vi "IrDA Date Server.vi"() -> ()   [LabVIEW 2013]
doc: "Sends the current time and date via TCP to all Date Client VIs that connect to it. This VI has two parts -- a loop that listens for each client to connect, and a loop that sends the date and time to each connection in the queue."
panel:
  in  "listen halted":bool
  in  "stop":bool
  out "# connections":i32
  in  "empty":refnum<k19>[](array[refnum])
  in  "empty":refnum<k19>[](array[refnum])
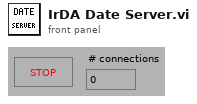
[diagram p1: front panel]
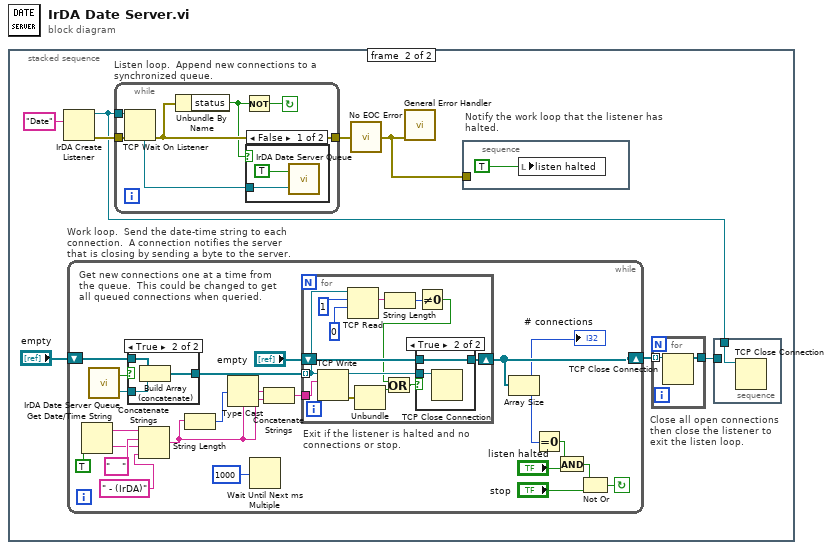
[diagram p0: block diagram]
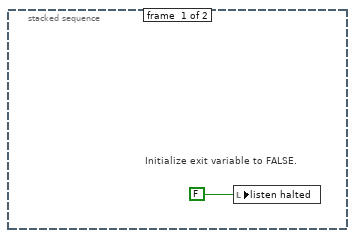
[diagram p2: hidden frame]
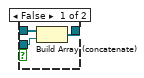
[diagram p3: hidden frame]
diagram:
  n1 = stacked-sequence {
    frame #0 {
      # "Initialize exit variable to FALSE."
      n2 = local write "listen halted"(FALSE) -> ()
    }
    frame #1 {
      # "Close all open connections then close the listener to exit the listen loop."
      # "Notify the work loop that the listener has halted."
      n3 = IrDA Create Listener(10:"Date" ("service name")) -> (0:w6:errorcluster, 3:w5:refnum<k19>)  [unwired: 1 in]
      n4 = while "Work loop.  Send the date-time string to each connection.  A connection notifies the server that is closing by sending a byte to the server." {
        shift-left: "empty" -> [w29]
        shift-right: [w20] -> w8
        stop <- w12 continue-if-true
        # "Get new connections one at a time from the queue.  This could be changed to get all queued connections when queried."
        # "Exit if the listener is halted and no connections or stop."
        n5 = Get Date/Time String(want seconds? (F)=TRUE) -> (date string=w25:string, time string=w17:string)  [unwired: 2 out]
        n6 = call "IrDA Date Server Queue.vi"() -> ("value"=w31:refnum<k19>, "valid?"=w30:bool)  [unwired: 2 in]
        n7 = case shown="True" w30 {
          tunnel: w31 -> [_ w53]
          tunnel: w29 -> [w50 w52]
          tunnel: [w50 w51] -> w27
          frame False {
          }
          frame True {
            n8 = Build Array (concatenate)(w52, w53) -> (w51:refnum<k19>[])
          }
        }
        n9 = Concatenate Strings(w25, "    ", w17, " - (IrDA)" ("string")) -> (w23:string)
        n10 = String Length(string=w23) -> (length=w24:i32)
        n11 = Type Cast(type=w23, x=w24) -> (*(type *) &x=w22:string)
        n12 = Wait Until Next ms Multiple(millisecond multiple=u32 1000) -> ()  [unwired: 1 out]
        n13 = Concatenate Strings(w22, w23) -> (w21:string)
        n14 = for {
          tunnel: w27 -> [w39] mode=indexing
          shift-right: [w40] -> w20
          shift-left: "empty" -> [w42]
          tunnel: w21 -> [w44]
          n15 = TCP Write(connection ID=w39, data in=w44) -> (connection ID out=w41:refnum<k19>, error out=w43:errorcluster)  [unwired: 1 in, 2 out]
          n16 = TCP Read(connection ID=w39, bytes to read=1, 9:0) -> (data out=w36:string)  [unwired: 1 in, 3 out]
          n17 = Unbundle(w43) -> ("status"=w33:bool)  [unwired: 2 out]
          n18 = String Length(string=w36) -> (length=w35:i32)
          n19 = Not Equal To 0?(x=w35) -> (x != 0?=w32:bool)
          n20 = Or(x=w32, y=w33) -> (x .or. y?=w34:bool)
          n21 = case shown="True" w34 {
            tunnel: w42 -> [w47 w49]
            tunnel: w41 -> [w46 w48]
            tunnel: [w45 w49] -> w40
            frame False {
              n22 = Build Array (concatenate)(w47, w46) -> (w45:refnum<k19>[])
            }
            frame True {
              n23 = TCP Close Connection(connection ID=w48) -> ()  [unwired: 1 in, 3 out]
            }
          }
        }
        n24 = Array Size(array=w20) -> (size(s)=w15:i32)
        "# connections" <- w15
        n25 = Equal To 0?(x=w15) -> (x = 0?=w16:bool)
        n26 = And(x=w16, y="listen halted") -> (x .and. y?=w13:bool)
        n27 = Not Or(1:"stop", 2:w13) -> (0:w12:bool)
      }
      n28 = while "Listen loop.  Append new connections to a synchronized queue." {
        tunnel: w5 -> [w57]
        tunnel: w6 -> [w58]
        tunnel: [w55] -> w4
        stop <- w59 continue-if-true
        n29 = TCP Wait On Listener(8:w58, 11:w57) -> (0:w55:errorcluster, 4:w56:refnum<k19>)  [unwired: 5 out]
        n30 = Unbundle By Name(w55) -> ("status"=w54:bool)
        n31 = Not(x=w54) -> (.not. x?=w59:bool)
        n32 = case shown="False" w54 {
          tunnel: w56 -> [w60 _]
          frame False {
            n33 = call "IrDA Date Server Queue.vi"("new value"=w60, "set queue? (F: de-queue)"=TRUE) -> ()  [unwired: 2 out]
          }
          frame True {
          }
        }
      }
      n34 = call "No EOC Error.vi"("error in"=w4) -> ("error out"=w3:errorcluster)  [unwired: 4 out]
      n35 = call <vilib>:"General Error Handler.vi"("error in (no error)"=w3) -> ()  [unwired: 1 in, 14 out]
      n36 = stacked-sequence {
        tunnel: w3 -> [_]
        frame #0 {
          n37 = local write "listen halted"(TRUE) -> ()
        }
      }
      n38 = for {
        tunnel: w8 -> [w63] mode=indexing
        tunnel: [w62] -> w9
        n39 = TCP Close Connection(connection ID=w63) -> (connection ID out=w62:refnum<k19>)  [unwired: 1 in, 2 out]
      }
      n40 = stacked-sequence {
        tunnel: w9 -> [_]
        tunnel: w5 -> [w64]
        frame #0 {
          n41 = TCP Close Connection(connection ID=w64) -> ()  [unwired: 1 in, 3 out]
        }
      }
    }
  }
